vi "Create_Dests.vi"(8 "error in (no error)":errorcluster, 11 "Class in":refnum<class "Installer.lvclass">) -> (0 "error out":errorcluster, 3 "Class out":refnum<class "Installer.lvclass">)   [LabVIEW 2020, in "Installer.lvclass"]
uses:
  <vilib>/AppBuilder/IB_Classes/Installer/Installer.lvclass
  <vilib>/AppBuilder/IB_Classes/Installer/Installer.lvclass/Installer.ctl
  <vilib>/AppBuilder/IB_Classes/Destination/IB_Destination.lvclass
  <vilib>/AppBuilder/IB_Classes/Dest_NI_NIPath/Dest_NI_NIPath.lvclass
  <vilib>/AppBuilder/IB_Classes/Destination/niLabel/niLabel.lvclass
  e:/builds/penguin/labview/branches/2020/dev/dist/vi.lib/AppBuilder/IB_Classes/Destination/niLabel/niLabel.lvclass
  e:/builds/penguin/labview/branches/2020/dev/dist/vi.lib/AppBuilder/IB_Classes/Destination/IB_Destination.lvclass
  e:/builds/penguin/labview/branches/2020/dev/dist/vi.lib/AppBuilder/IB_Classes/Dest_NI_NIPath/Dest_NI_NIPath.lvclass
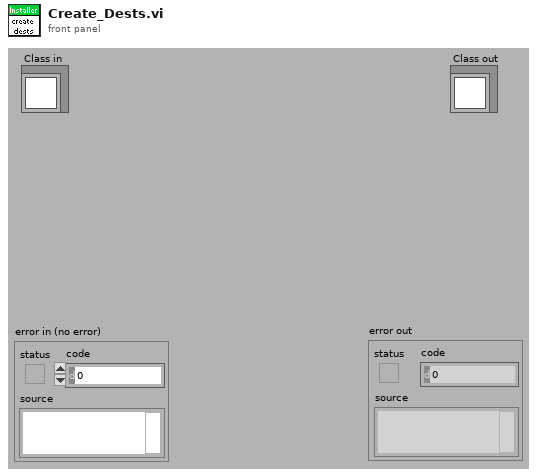
[diagram p1: front panel]
types:
  T1 = typedef "CDK_sTypeDef_AppBitness.ctl" = enum16{"invalid", "32-bit", "64-bit"}
  T2 = typedef "IB_Dest_niLabel.ctl" = cluster{"local path":path}
  T3 = typedef "IB_Destination.ctl" = cluster{"name":string, "unlock":bool, "parentTag":string, "destTag":string, "eng_installPath":string}
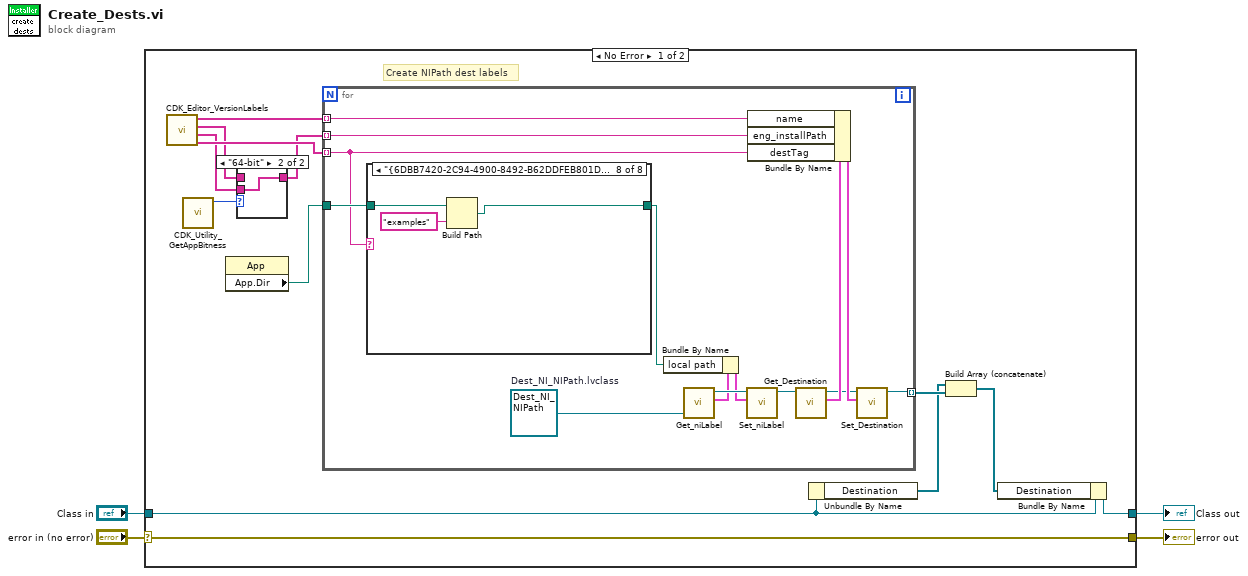
[diagram p0: block diagram]
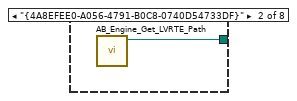
[diagram p4: hidden frame]
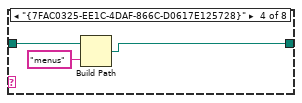
[diagram p6: hidden frame]
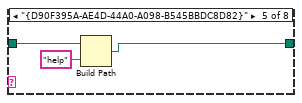
[diagram p7: hidden frame]
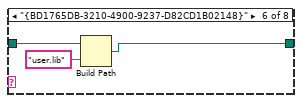
[diagram p8: hidden frame]
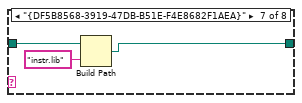
[diagram p9: hidden frame]
diagram:
  n1 = case shown="No Error" "error in (no error)" {
    selector: "error in (no error)" -> [w12 w52]
    tunnel: "Class in" -> [w15 w53]
    tunnel: [w13 w53] -> w3
    tunnel: [w12 w52] -> w1
    frame No Error {
      # "Create NIPath dest labels"
      n2 = call <resource>:"CDK_Editor_VersionLabels.vi"() -> ("DNL_NIPath guids"=w11:string[], "DNL_NIPath labels 64-bit"=w8:string[], "DNL_NIPath labels 32-bit"=w7:string[], "NIPath aliases"=w9:string[])  [unwired: 8 in]
      n3 = call <resource>:"CDK_Utility_GetAppBitness.vi"() -> ("app bitness"=w10:T1)  [unwired: 11 out]
      n4 = property class="App"() -> ("App.Dir"=w5:path)  [unwired: 2 in, 2 out]
      n5 = case shown="\"64-bit\"" w10 {
        tunnel: w8 -> [_ w19]
        tunnel: [w18 w19] -> w6
        tunnel: w7 -> [w18 _]
        frame "32-bit", Default {
        }
        frame "64-bit" {
        }
      }
      n6 = for {
        tunnel: w9 -> [w23] mode=indexing
        tunnel: [w27] -> w17 mode=indexing
        tunnel: w11 -> [w20] mode=indexing
        tunnel: w6 -> [w30] mode=indexing
        tunnel: w5 -> [w21]
        w29 = refnum<class "Dest_NI_NIPath.lvclass"> refnum  # Dest_NI_NIPath.lvclass
        n7 = case shown="\"{6DBB7420-2C94-4900-8492-B62DDFEB801D}\"" w20 {
          tunnel: [w34 w35 w36 w37 w40 w43 w46 w49] -> w22
          tunnel: w21 -> [w34 _ w36 w39 w42 w45 w48 w51]
          frame Default {
          }
          frame "{4A8EFEE0-A056-4791-B0C8-0740D54733DF}" {
            n8 = call <vilib>:"AB_Engine_Get_LVRTE_Path.vi"() -> ("Run-Time Engine Path"=w35:path)  [unwired: 9 in, 2 out]
          }
          frame "{E20B5188-6575-4366-9109-D4EA9AB7500C}" {
          }
          frame "{7FAC0325-EE1C-4DAF-866C-D0617E125728}" {
            n9 = Build Path(base path=w39, name or relative path="menus") -> (appended path=w37:path)
          }
          frame "{D90F395A-AE4D-44A0-A098-B545BBDC8D82}" {
            n10 = Build Path(base path=w42, name or relative path="help") -> (appended path=w40:path)
          }
          frame "{BD1765DB-3210-4900-9237-D82CD1B02148}" {
            n11 = Build Path(base path=w45, name or relative path="user.lib") -> (appended path=w43:path)
          }
          frame "{DF5B8568-3919-47DB-B51E-F4E8682F1AEA}" {
            n12 = Build Path(base path=w48, name or relative path="instr.lib") -> (appended path=w46:path)
          }
          frame "{6DBB7420-2C94-4900-8492-B62DDFEB801D}" {
            n13 = Build Path(base path=w51, name or relative path="examples") -> (appended path=w49:path)
          }
        }
        n14 = call <vilib>:"Get_niLabel.vi"("niLabel in"=w29) -> ("data"=w25:T2, "niLabel out"=w26:refnum<class "Dest_NI_NIPath.lvclass">)  [unwired: 8 in, 1 out]
        n15 = Bundle By Name(cluster=w25, "local path"=w22) -> (w24:T2)
        n16 = call <vilib>:"Set_niLabel.vi"("data"=w24, "niLabel in"=w26) -> ("niLabel out"=w28:refnum<class "Dest_NI_NIPath.lvclass">)  [unwired: 8 in, 1 out]
        n17 = call <vilib>:"Get_Destination.vi"("IB_Destination in"=w28) -> ("data"=w33:T3, "IB_Destination out"=w31:refnum<class "Dest_NI_NIPath.lvclass">)  [unwired: 8 in, 1 out]
        n18 = Bundle By Name(cluster=w33, "name"=w23, "eng_installPath"=w30, "destTag"=w20) -> (w32:T3)
        n19 = call <vilib>:"Set_Destination.vi"("data"=w32, "IB_Destination in"=w31) -> ("IB_Destination out"=w27:refnum<class "Dest_NI_NIPath.lvclass">)  [unwired: 8 in, 1 out]
      }
      n20 = Unbundle By Name(w15) -> ("Destination"=w14:refnum<class "IB_Destination.lvclass">[])
      n21 = Build Array (concatenate)(w14, w17) -> (w16:refnum<class "IB_Destination.lvclass">[])
      n22 = Bundle By Name(cluster=w15, "Destination"=w16) -> (w13:refnum<class "Installer.lvclass">)
    }
    frame Error {
    }
  }
  "error out" <- w1
  "Class out" <- w3
